vi "WebSocket Client Handshake.vi"(4 "remote port or service name":u16=7890, 6 "address":string="localhost", 8 "error in (no error)":errorcluster, 9 "timeout ms (1000)":i32=1000, 11 "WebSocket Connection in":refnum<k5>) -> (0 "error out":errorcluster, 2 "Return Headers Out":variant, 3 "WebSocket Connection out":refnum<k5>)   [LabVIEW 2018]
doc: "Performs a client-side handshake. Sends the initial handshake HTTP header and waits for response from WebSocket server. Validates received accept key from the response.\nWebSockets API 1.3.0.13\nSam Sharp - Intelligent Energy\nCopyright (c) 2015, Intelligent Energy"
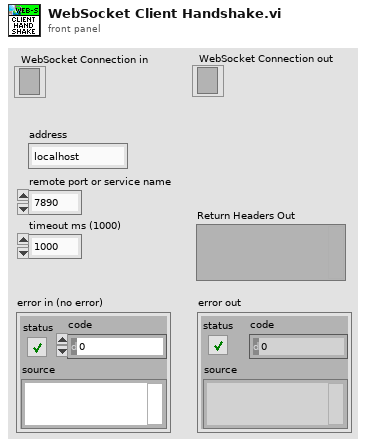
[diagram p1: front panel]
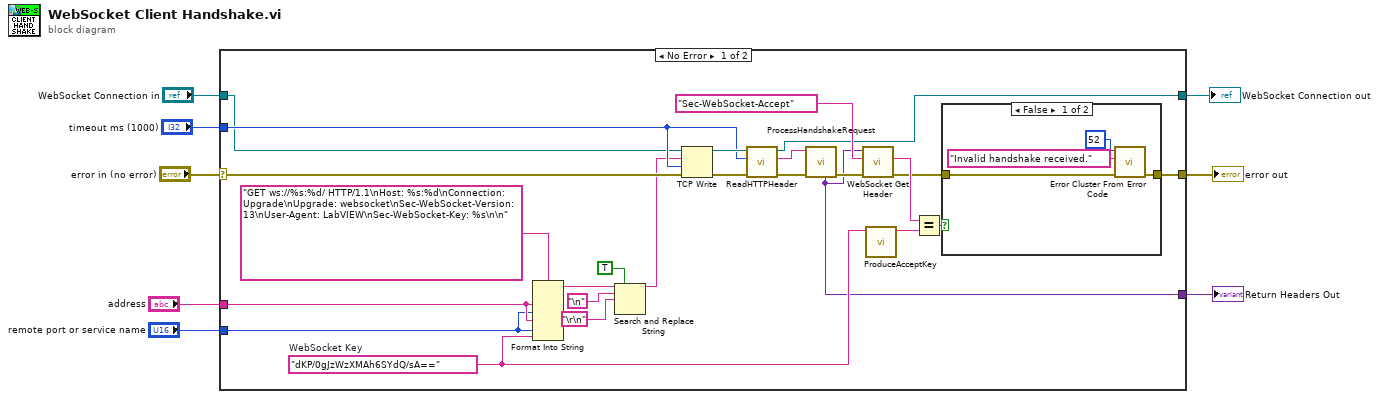
[diagram p0: block diagram]
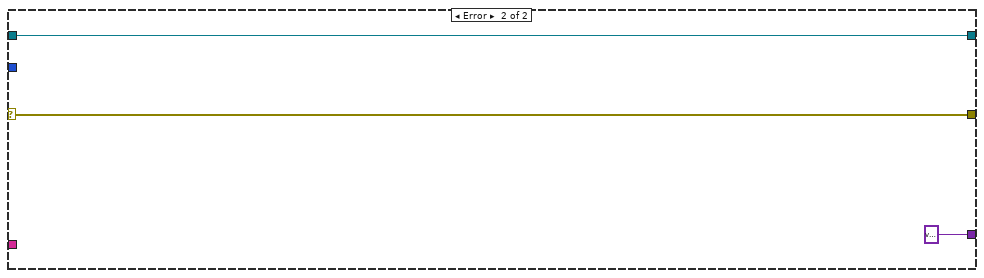
[diagram p3: hidden frame]
diagram:
  n1 = case shown="No Error" "error in (no error)" {
    selector: "error in (no error)" -> [w31 w41]
    tunnel: [w13 w40] -> w8
    tunnel: "WebSocket Connection in" -> [w9 w40]
    tunnel: [w10 w41] -> w5
    tunnel: "timeout ms (1000)" -> [w28 _]
    tunnel: [w15 variant ("Headers Out")] -> w3
    tunnel: "address" -> [w21 _]
    tunnel: "remote port or service name" -> [w20 _]
    frame No Error {
      w19 = "dKP/0gJzWzXMAh6SYdQ/sA=="  # WebSocket Key
      n2 = Format Into String(format string="GET ws://%s:%d/ HTTP/1.1\nHost: %s:%d\nConnection: Upgrade\nUpgrade: websocket\nSec-WebSocket-Version: 13\nUser-Agent: LabVIEW\nSec-WebSocket-Key: %s\n\n", w21, w20, w21, w20, w19) -> (resulting string=w23:string)  [unwired: 2 in, 1 out]
      n3 = Search and Replace String(replace all?=TRUE ("replace all? (F)"), input string=w23, search string="\n", replace string="\r\n") -> (result string=w27:string)  [unwired: 4 in, 3 out]
      n4 = TCP Write(connection ID=w9, data in=w27, error in (no error)=w31, 9:w28) -> (connection ID out=w32:refnum<k5>, error out=w33:errorcluster)  [unwired: 1 out]
      n5 = call "ReadHTTPHeader.vi"("error in (no error)"=w33, "timeout ms (25000)"=w28, "WebSocket Connection in"=w32) -> ("error out"=w14:errorcluster, "HTTP Header"=w24:string, "WebSocket Connection out"=w13:refnum<k5>)  [unwired: 6 in]
      n6 = call "ProcessHandshakeRequest.vi"("error in (no error)"=w14, "HTTP Headers"=w24) -> ("error out"=w18:errorcluster, "Headers Out"=w15:variant)  [unwired: 4 in, 4 out]
      n7 = call "WebSocket Get Header.vi"("error in (no error)"=w18, "Name"="Sec-WebSocket-Accept", "Headers In"=w15) -> ("error out"=w11:errorcluster, "Data"=w16:string)  [unwired: 5 in, 2 out]
      n8 = call "ProduceAcceptKey.vi"("Sec-WebSocket-Key"=w19) -> ("Sec-WebSocket-Accept"=w25:string)  [unwired: 10 in]
      n9 = Equal?(x=w16, y=w25) -> (x = y?=w12:bool)
      n10 = case shown="False" w12 {
        tunnel: w11 -> [w36 w38]
        tunnel: [w37 w38] -> w10
        frame False {
          n11 = call <vilib>:"Error Cluster From Error Code.vi"("error in (no error)"=w36, "error message (\"\")"="Invalid handshake received." ("error message (\"\")"), "error code (0)"=52) -> ("error out"=w37:errorcluster)  [unwired: 6 in]
        }
        frame True {
        }
      }
    }
    frame Error {
    }
  }
  "WebSocket Connection out" <- w8
  "error out" <- w5
  "Return Headers Out" <- w3
